vi "VIPInstall.vi"() -> ()   [LabVIEW 2015, in "G CLI VIP.lvlib"]
uses:
  G CLI VIP.lvlib
  <vilib>/Wiresmith Technology/G CLI/CLI Class/CLI.lvclass
  <vilib>/JKI/VIPM API/VIPM API_vipm_api.lvlib
panel:
  out "error out":errorcluster
  # "VIP Install"
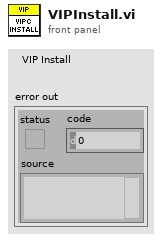
[diagram p1: front panel]
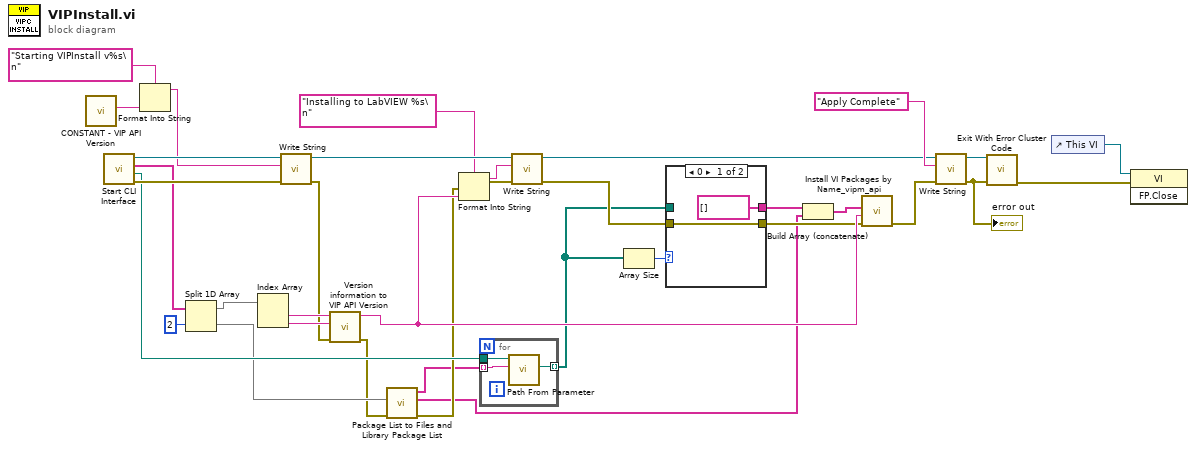
[diagram p0: block diagram]
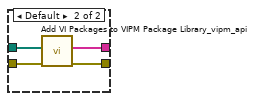
[diagram p2: hidden frame]
diagram:
  n1 = call "CONSTANT - VIP API Version.vi"() -> ("Version"=w32:string)  [unwired: 11 in]
  n2 = call <vilib>:"Start CLI Interface.vi"() -> ("error out"=w34:errorcluster, "Working Directory"=w26:path, "Custom Parameters"=w11:string[], "CLI out"=w35:refnum<class "CLI.lvclass">)  [unwired: 8 in]
  n3 = Format Into String(format string="Starting VIPInstall v%s\n", w32) -> (resulting string=w31:string)  [unwired: 2 in, 1 out]
  n4 = Split 1D Array(array=w11, index=2) -> (first subarray=w9:string[], second subarray=w8:string[])
  n5 = Index Array(array=w9) -> (element #1=w29:string, element #2=w28:string)  [unwired: 2 in]
  n6 = call <vilib>:"Write String.vi"("error in (no error)"=w34, "Text to Write"=w31, "CLI in"=w35) -> ("error out"=w27:errorcluster, "CLI out"=w20:refnum<class "CLI.lvclass">)  [unwired: 7 in]
  n7 = call "Version information to VIP API Version.vi"("error in (no error)"=w27, "Bitness String"=w28, "Version String"=w29) -> ("error out"=w7:errorcluster, "VIP Version"=w15:string)  [unwired: 7 in]
  n8 = call "Package List to Files and Library Package List.vi"("error in (no error)"=w7, "Packages"=w8) -> ("error out"=w6:errorcluster, "Library Packages"=w3:string[], "File Packages"=w5:string[])  [unwired: 7 in]
  n9 = Format Into String(format string="Installing to LabVIEW %s\n", error in=w6, w15) -> (resulting string=w16:string, error out=w18:errorcluster)  [unwired: 1 in]
  n10 = for {
    tunnel: w26 -> [w38]
    tunnel: [w37] -> w2 mode=indexing
    tunnel: w5 -> [w36] mode=indexing
    n11 = call <vilib>:"Path From Parameter.vi"("Path Parameter"=w36, "Working Directory"=w38) -> ("Full Path"=w37:path)  [unwired: 9 in]
  }
  n12 = call <vilib>:"Write String.vi"("error in (no error)"=w18, "Text to Write"=w16, "CLI in"=w20) -> ("error out"=w12:errorcluster, "CLI out"=w19:refnum<class "CLI.lvclass">)  [unwired: 7 in]
  n13 = Array Size(array=w2) -> (size(s)=w1:i32)
  n14 = case shown="0" w1 {
    tunnel: [string[] [] ("Package Names Added") w44] -> w14
    tunnel: [w40 w43] -> w13
    tunnel: w12 -> [w40 w42]
    tunnel: w2 -> [_ w41]
    frame 0 {
    }
    frame Default {
      n15 = call <vilib>:"Add VI Packages to VIPM Package Library_vipm_api.vi"("error in (no error)"=w42, "Packages to add to VIPM Library (vipc,vip,ogp)"=w41) -> ("error out"=w43:errorcluster, "Package Names Added"=w44:string[])  [unwired: 8 in]
    }
  }
  n16 = Build Array (concatenate)(w14, w3) -> (w4:string[])
  n17 = call <vilib>:"Install VI Packages by Name_vipm_api.vi"("error in (no error)"=w13, "LabVIEW Version"=w15, "Package Names to Install []"=w4) -> ("error out"=w30:errorcluster)  [unwired: 8 in]
  n18 = call <vilib>:"Write String.vi"("error in (no error)"=w30, "Text to Write"="Apply Complete", "CLI in"=w19) -> ("error out"=w25:errorcluster, "CLI out"=w24:refnum<class "CLI.lvclass">)  [unwired: 7 in]
  "error out" <- w25
  n19 = call <vilib>:"Exit With Error Cluster Code.vi"("error in (no error)"=w25, "CLI in"=w24) -> ("error out"=w22:errorcluster)  [unwired: 9 in]
  n20 = control-ref of="This VI"() -> (w21:refnum<vi>)
  n21 = invoke class="VI" method="FP.Close"(reference=w21, error in=w22) -> ()  [unwired: 1 in, 3 out]
